vi "侧铆试验判定.vi"(7 "Result":refnum<vi>, 10 "判定参数":T1, 11 "XY曲线":cluster{"X":dbl[], "Y":dbl[]}[](array[cluster])) -> (2 "判定项长度":i32, 3 "OK？":bool)   [LabVIEW 2020]
uses:
  Global_Variable/Global.vi
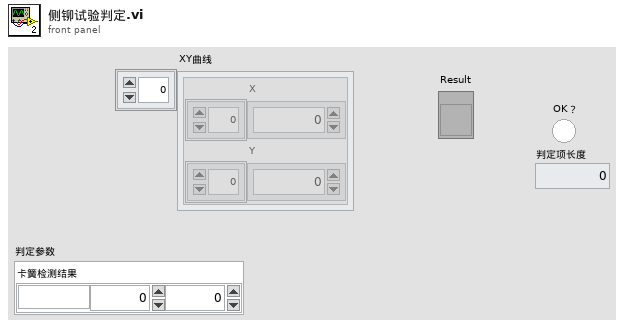
[diagram p1: front panel]
types:
  T1 = cluster{"卡簧检测结果":cluster{"单位":string, "下限":dbl, "上限":dbl}}
  T2 = cluster{"相机结果":dbl, "相机结果1":sgl, "工装移载位移":sgl, "电缸位移":sgl, "输入扭矩":sgl, "输出扭矩(小)":sgl, "输出扭矩(大)":sgl, "电缸压力":sgl}
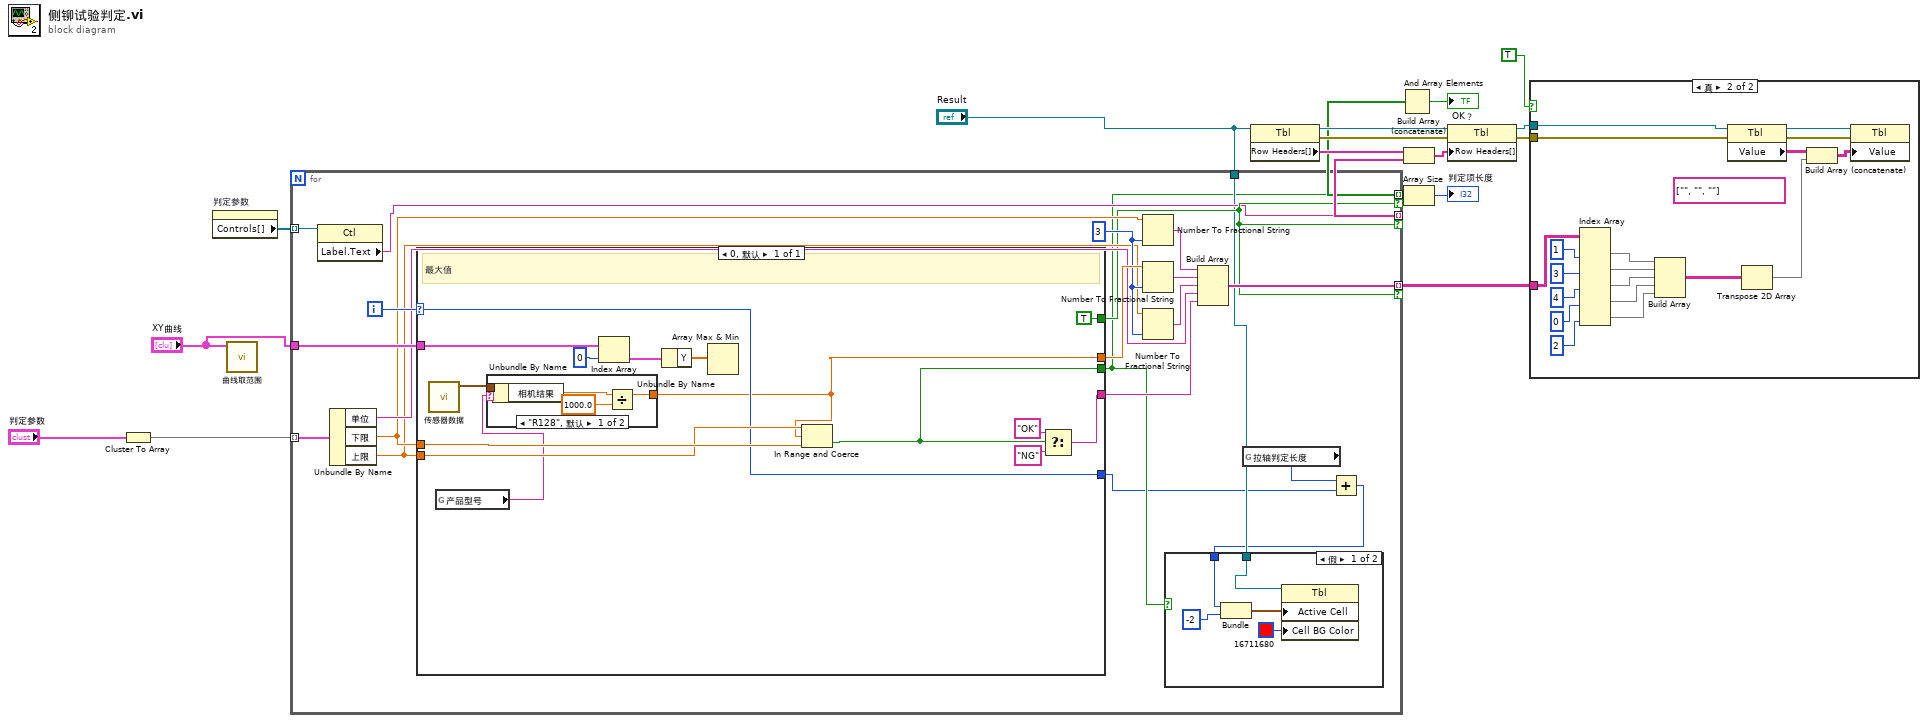
[diagram p0: block diagram]
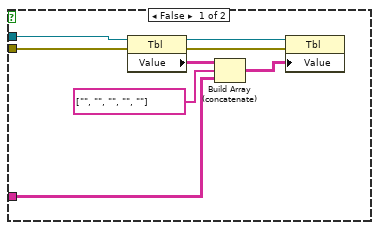
[diagram p2: hidden frame]
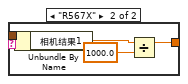
[diagram p4: hidden frame]
diagram:
  n1 = Cluster To Array(cluster="判定参数") -> (array=w17:cluster{"单位":string, "下限":dbl, "上限":dbl}[])
  n2 = property on="判定参数" class="Clust (严格)"() -> ("Controls[]"=w7:refnum<vi>[])  [unwired: 2 in, 2 out]
  n3 = call "曲线取范围.vi"("曲线In"="XY曲线") -> ()  [unwired: 10 in, 1 out]
  n4 = for {
    tunnel: w17 -> [w38] mode=indexing
    tunnel: w7 -> [w36] mode=indexing
    tunnel: "XY曲线" -> [w34]
    tunnel: [w21] -> w5 mode=indexing if=w24
    tunnel: [w25] -> w8 mode=indexing if=w24
    tunnel: [w23] -> w10 mode=indexing if=w24
    tunnel: "Result" -> [w22]
    i -> [w37]
    w33 = i16 3 ("精度(6)")
    n5 = property class="Ctl"(reference=w36) -> ("Label.Text"=w23:string)  [unwired: 1 in, 2 out]
    n6 = Unbundle By Name(w38) -> ("单位"=w28:string, "下限"=w27:dbl, "上限"=w26:dbl)
    n7 = case shown="0, 默认" w37 {
      selector: w37 -> [w48]
      tunnel: [w46] -> w35
      tunnel: w34 -> [w58]
      tunnel: [w53] -> w29
      tunnel: [w44] -> w21
      tunnel: w27 -> [w52]
      tunnel: w26 -> [w51]
      tunnel: [TRUE] -> w24
      tunnel: [w48] -> w20
      frame 0, Default {
        # "最大值"
        n8 = call "传感器数据.vi"() -> ("传感器读数"=w47:T2)  [unwired: 11 in]
        n9 = global read "Global.vi" "产品型号"() -> (w45:string)
        n10 = case shown="\"R128\", 默认" w45 {
          tunnel: w47 -> [w62 w66]
          tunnel: [w60 w64] -> w46
          frame "R128", Default {
            n11 = Unbundle By Name(w62) -> ("相机结果"=w61:dbl)
            n12 = Divide(x=w61, y=sgl 1000.0) -> (x/y=w60:dbl)
          }
          frame "R567X" {
            n13 = Unbundle By Name(w66) -> ("相机结果1"=w65:sgl)
            n14 = Divide(x=w65, y=sgl 1000.0) -> (x/y=w64:sgl)
          }
        }
        n15 = Index Array(array=w58, index=0 ("索引")) -> (element=w56:cluster{"X":dbl[], "Y":dbl[]})
        n16 = Unbundle By Name(w56) -> ("Y"=w49:dbl[])
        n17 = Array Max & Min(array=w49) -> ()  [unwired: 4 out]
        n18 = In Range and Coerce(upper limit=w51, x=w46, lower limit=w52) -> (In Range?=w44:bool)  [unwired: 1 out]
        n19 = Select(t="OK", s=w44, f="NG") -> (s? t:f=w53:string)
      }
    }
    n20 = Number To Fractional String(number=w27, precision (6)=w33) -> (F-format string=w32:string)  [unwired: 2 in]
    n21 = Number To Fractional String(number=w35, precision (6)=w33) -> (F-format string=w31:string)  [unwired: 2 in]
    n22 = Number To Fractional String(number=w26, precision (6)=w33) -> (F-format string=w30:string)  [unwired: 2 in]
    n23 = Build Array(w32, w31, w30, w28, w29) -> (w25:string[])
    n24 = global read "判定参数.vi" "拉轴判定长度"() -> (w18:i32)
    n25 = Add(x=w18, y=w20) -> (x+y=w19:i32)
    n26 = case shown="假" w21 {
      tunnel: w22 -> [w43 _]
      tunnel: w19 -> [w39 _]
      frame False {
        n27 = Bundle(w39, "索引"=-2) -> (w40:cluster{i32, "索引":i32})  [unwired: 1 in]
        n28 = property class="Tbl"(reference=w43, "Active Cell"=w40, "Cell BG Color"=u32 16711680 ("活动单元格:单元格背景色")) -> ()  [unwired: 1 in, 2 out]
      }
      frame True {
      }
    }
  }
  n29 = property class="Tbl"(reference="Result") -> (reference out=w12:refnum<vi>, error out=w15:errorcluster, "Row Headers[]"=w9:string[])  [unwired: 1 in]
  n30 = And Array Elements(Boolean array=w5) -> (logical AND=→"OK？":bool)
  n31 = Build Array (concatenate)(w9, w10) -> (w11:string[])
  n32 = Array Size(array=w5) -> (size(s)=→"判定项长度":i32)
  n33 = property class="Tbl"(reference=w12, error in=w15, "Row Headers[]"=w11) -> (reference out=w13:refnum<vi>, error out=w14:errorcluster)
  n34 = case shown="真" TRUE {
    tunnel: w14 -> [w72 w91]
    tunnel: w13 -> [w69 w88]
    tunnel: w8 -> [w68 w80]
    frame False {
      n35 = property class="Tbl"(reference=w69, error in=w72) -> (reference out=w70:refnum<vi>, error out=w71:errorcluster, "Value"=w73:string[][])
      n36 = Build Array (concatenate)(w73, string[] ["", "", "", "", ""], w68) -> (w74:string[][])
      n37 = property class="Tbl"(reference=w70, error in=w71, "Value"=w74) -> ()  [unwired: 2 out]
    }
    frame True {
      (unwired) string[] ["", "", ""]
      n38 = Index Array(array=w80, index (col) #1=1 ("禁用的索引 (列)"), index (col) #2=3 ("索引 (列)"), index (col) #3=4 ("索引 (列)"), index (col) #4=0 ("索引 (列)"), index (col) #5=2 ("索引 (列)")) -> (element #1=w84:string[], element #2=w85:string[], element #3=w86:string[], element #4=w76:string[], element #5=w75:string[])  [unwired: 5 in]
      n39 = Build Array(w84, w85, w86, w76, w75) -> (w87:string[][])
      n40 = property class="Tbl"(reference=w88, error in=w91) -> (reference out=w89:refnum<vi>, error out=w90:errorcluster, "Value"=w92:string[][])
      n41 = Transpose 2D Array(2D array=w87) -> (transposed array=w79:string[][])
      n42 = Build Array (concatenate)(w92, w79) -> (w93:string[][])
      n43 = property class="Tbl"(reference=w89, error in=w90, "Value"=w93) -> ()  [unwired: 2 out]
    }
  }
